vi "GetPowerSpectrum.vi"(8 "error in (no error)":errorcluster, 10 "FftData in":csg[](array[numeric]), 11 "SETI_LV_FPGA in":refnum<class "SETI_LV_FPGA.lvclass">) -> (0 "error out":errorcluster, 2 "PowerSpectrum out":sgl[](array[numeric]), 3 "SETI_LV_FPGA out":refnum<class "SETI_LV_FPGA.lvclass">)   [LabVIEW 2015, in "SETI_LV_FPGA.lvclass"]
uses:
  SETI_LV_FPGA.lvclass
  SETI_LV/SETI_LV.lvlib
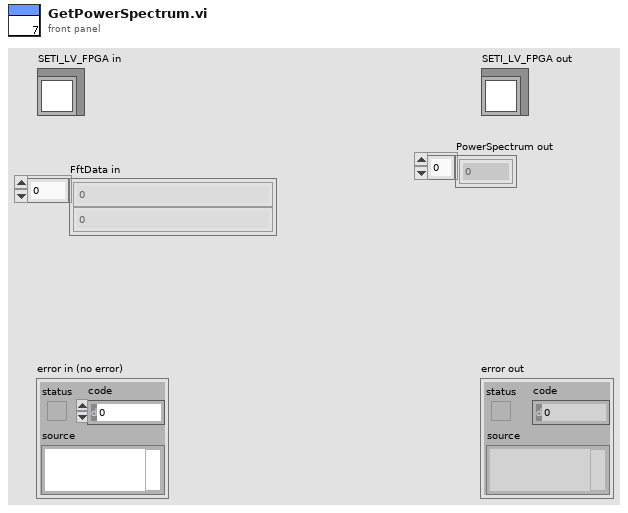
[diagram p1: front panel]
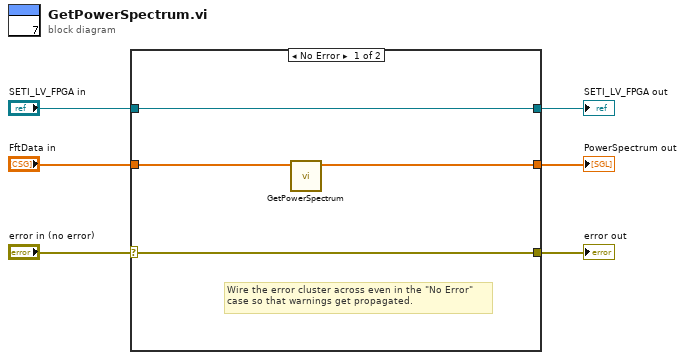
[diagram p0: block diagram]
diagram:
  n1 = case shown="No Error" "error in (no error)" {
    selector: "error in (no error)" -> [w9 w13]
    tunnel: [w9 w13] -> w5
    tunnel: [w10 w12] -> w3
    tunnel: "SETI_LV_FPGA in" -> [w10 w12]
    tunnel: "FftData in" -> [w8 w11]
    tunnel: [w7 w11] -> w1
    frame No Error {
      # "Wire the error cluster across even in the \"No Error\"\ncase so that warnings get propagated."
      n2 = call "GetPowerSpectrum.vi"("Fft Results (in)"=w8) -> ("PowerSpectrum (out)"=w7:sgl[])  [unwired: 10 in]
    }
    frame Error {
    }
  }
  "error out" <- w5
  "SETI_LV_FPGA out" <- w3
  "PowerSpectrum out" <- w1
